vi "SSC DCPower Configure Voltage Sequence.vi"(0 "DCPower SSC in":T1[](array[typedef]), 5 "Voltage Level Start":dbl, 7 "Voltage Step":dbl=1.0 min=1.0, 9 "Voltage Level Stop":dbl, 11 "error in":errorcluster) -> (4 "DCPower SSC out":T1[](array[typedef]), 15 "error out":errorcluster)   [LabVIEW 2019]
doc: "This VI configures the Voltage Level in Sequence\nIt can generate volt from low to high and vice versa"
uses:
  Instrument Control/DCPower/SSC DCPower/SSC DCPower.ctl
  <vilib>/Analysis/1siggen.llb/Ramp Pattern by Delta.vi
  <vilib>/Analysis/NI_AALBase.lvlib
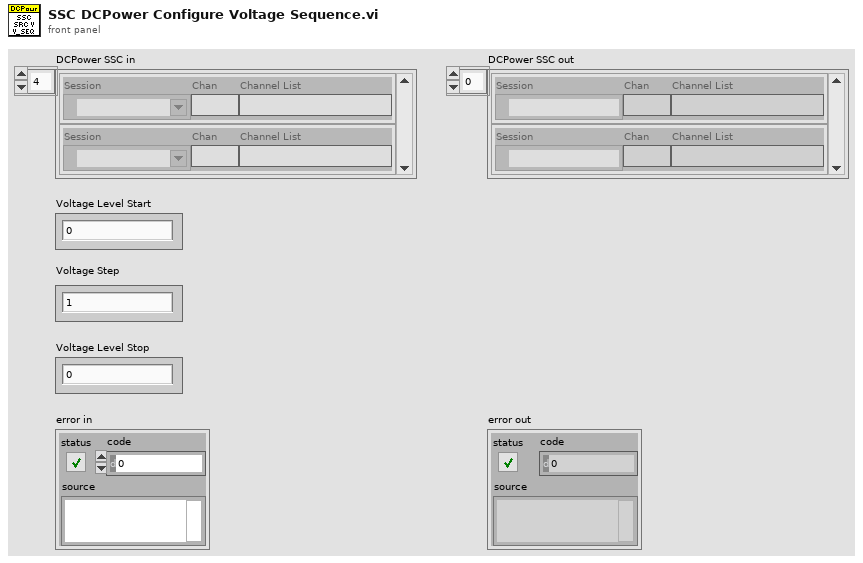
[diagram p1: front panel]
types:
  T1 = typedef "SSC DCPower.ctl" = cluster{"Session":refnum<k15>, "Chan":string, "Channel List":string}
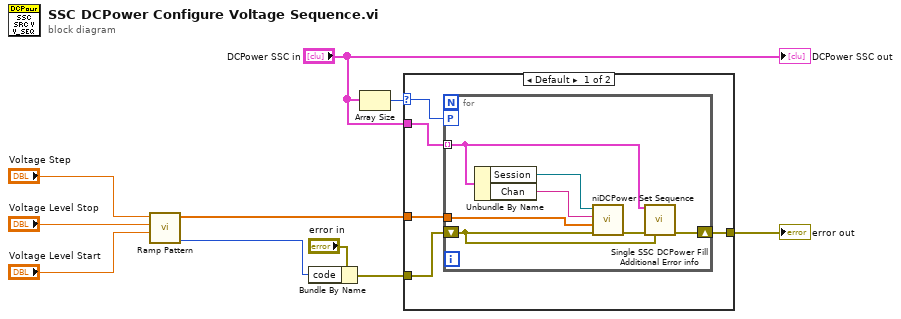
[diagram p0: block diagram]
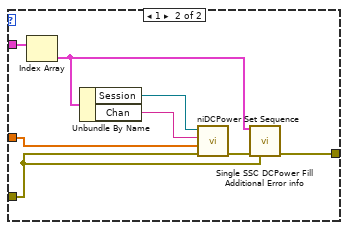
[diagram p2: hidden frame]
diagram:
  n1 = call-poly <vilib>:"Ramp Pattern.vi"("start"="Voltage Level Start", "end"="Voltage Level Stop", "delta"="Voltage Step") -> ("error"=w2:i32, "Ramp Pattern"=w7:dbl[])  [unwired: 6 in, 1 out]
  n2 = Bundle By Name(cluster="error in", "code"=w2) -> (w1:errorcluster)
  n3 = Array Size(array="DCPower SSC in") -> (size(s)=w9:i32)
  n4 = case shown="Default" w9 {
    selector: w9 -> [w13 _]
    tunnel: [w15 w30] -> w10
    tunnel: w1 -> [w14 w29]
    tunnel: "DCPower SSC in" -> [w12 w28]
    tunnel: w7 -> [w11 w23]
    frame Default {
      n5 = for {
        tunnel: w12 -> [w19] mode=indexing
        workers-P: w13 -> [_]
        shift-right: [w20] -> w15
        shift-left: w14 -> [w16]
        tunnel: w11 -> [w18]
        n6 = Unbundle By Name(w19) -> ("Session"=w22:refnum<k15>, "Chan"=w21:string)
        n7 = call <instrlib>:"niDCPower Set Sequence.vi"("error in (no error)"=w16, "values"=w18, "channel name"=w21, "instrument handle"=w22) -> ("error out"=w17:errorcluster)  [unwired: 6 in, 1 out]
        n8 = call "Single SSC DCPower Fill Additional Error info.vi"("DCPower SSC in"=w19, "error in"=w17, "previous error in"=w16) -> ("error out"=w20:errorcluster)  [unwired: 12 in]
      }
    }
    frame 1 {
      n9 = Index Array(array=w28) -> (element=w24:T1)  [unwired: 1 in]
      n10 = Unbundle By Name(w24) -> ("Session"=w26:refnum<k15>, "Chan"=w25:string)
      n11 = call <instrlib>:"niDCPower Set Sequence.vi"("error in (no error)"=w29, "values"=w23, "channel name"=w25, "instrument handle"=w26) -> ("error out"=w27:errorcluster)  [unwired: 6 in, 1 out]
      n12 = call "Single SSC DCPower Fill Additional Error info.vi"("DCPower SSC in"=w24, "error in"=w27, "previous error in"=w29) -> ("error out"=w30:errorcluster)  [unwired: 12 in]
    }
  }
  "error out" <- w10
  "DCPower SSC out" <- "DCPower SSC in"
